vi "Read Target Name.vi"(8 "error in (no error)":errorcluster, 11 "myRIOMetaDataObj in":refnum<class "myRIOMetaDataObj.lvclass">) -> (0 "error out":errorcluster, 2 "Target Name":string="myRIO Target", 3 "myRIOMetaDataObj out":refnum<class "myRIOMetaDataObj.lvclass">)   [LabVIEW 2021, in "myRIOMetaDataObj.lvclass"]
uses:
  myRIOMetaDataObj.lvclass
  myRIOMetaDataObj.lvclass/myRIOMetaDataObj.ctl
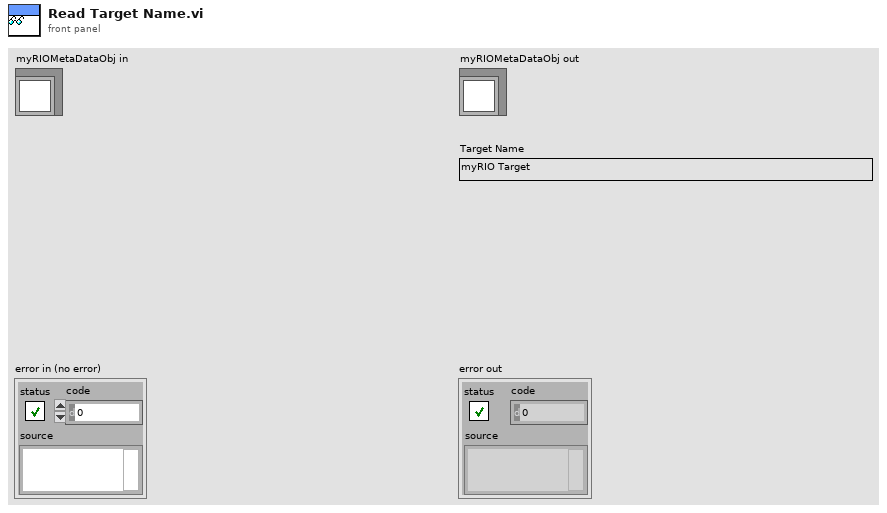
[diagram p1: front panel]
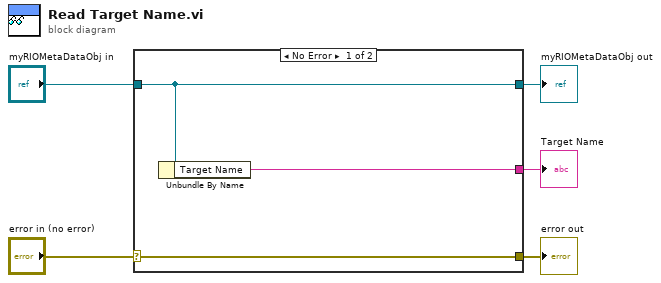
[diagram p0: block diagram]
diagram:
  n1 = case shown="No Error" "error in (no error)" {
    selector: "error in (no error)" -> [w8 w9]
    tunnel: [w8 w9] -> w4
    tunnel: [w7 w10] -> w2
    tunnel: "myRIOMetaDataObj in" -> [w7 w10]
    tunnel: [w6 _] -> w1
    frame No Error {
      n2 = Unbundle By Name(w7) -> ("Target Name"=w6:string)
    }
    frame Error {
    }
  }
  "error out" <- w4
  "myRIOMetaDataObj out" <- w2
  "Target Name" <- w1
